vi "browse.vi"(7 "LabVIEW Web Service Request":refnum<class "Web Request.lvclass">) -> ()   [LabVIEW 2024]
uses:
  <vilib>/wsapi/Web Request.lvclass
  <vilib>/Utility/error.llb/Trim Whitespace One-Sided.vi
panel:
  # "Use the Web Service Request input terminal to call the VIs on the Web Services palette. Do not remove it from the connector pane unless you don't need access to the palette."
  # "Each additional control wired to the connector pane will be available as an input in the URL. To include an indicator in terminal-mode output (the default setting), it must also be wired to the connector pane."
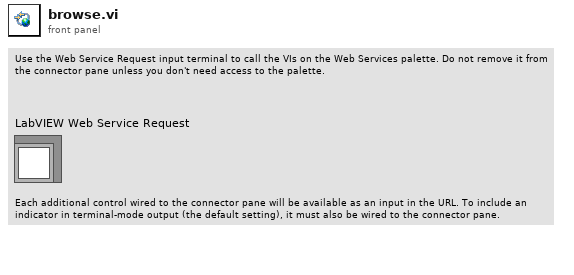
[diagram p1: front panel]
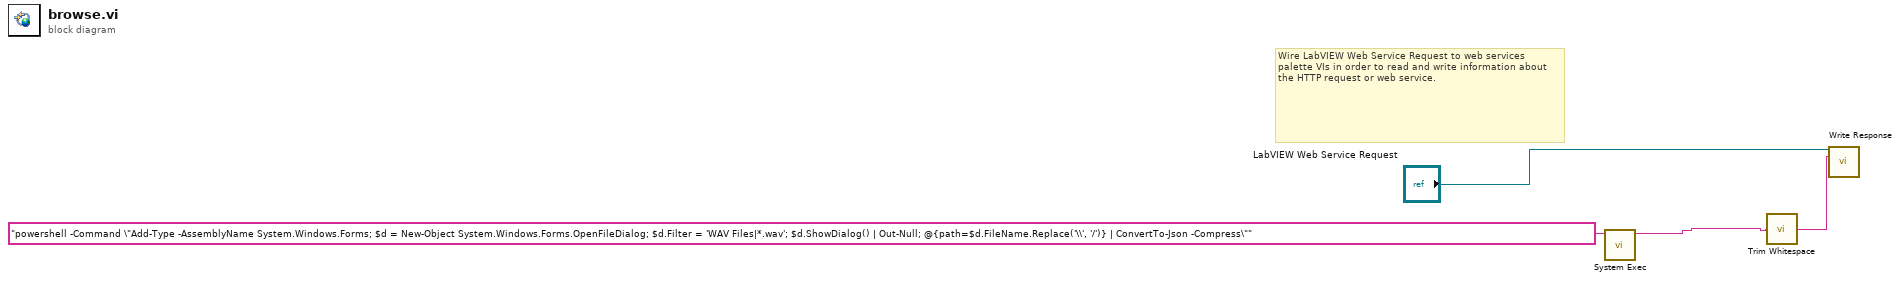
[diagram p0: block diagram]
diagram:
  # "Wire LabVIEW Web Service Request to web services palette VIs in order to read and write information about the HTTP request or web service."
  n1 = call <vilib>:"System Exec.vi"("command line"="powershell -Command \"Add-Type -AssemblyName System.Windows.Forms; $d = New-Object System.Windows.Forms.OpenFileDialog; $d.Filter = 'WAV Files|*.wav'; $d.ShowDialog() | Out-Null; @{path=$d.FileName.Replace('\\', '/')} | ConvertTo-Json -Compress\"") -> ("standard output"=w1:string)  [unwired: 7 in, 3 out]
  n2 = call <vilib>:"Trim Whitespace.vi"("string"=w1) -> ("trimmed string"=w2:string)  [unwired: 1 in]
  n3 = call <vilib>:"Write Response.vi"("LabVIEW Web Service Request"="LabVIEW Web Service Request", "response string"=w2) -> ()  [unwired: 12 in, 2 out]
